vi "ReserveMemory.vi"(8 "error in (no error)":errorcluster, 10 "#DGs":i32=1, 11 "BME_DG_System in":refnum<class "BME_DG_System.lvclass">) -> (0 "error out":errorcluster, 3 "BME_DG_System out":refnum<class "BME_DG_System.lvclass">)   [LabVIEW 2009, in "BME_DG_System.lvclass"]
uses:
  BME_DG_System.lvclass
  BME_DG_System.lvclass/BME_DG_System.ctl
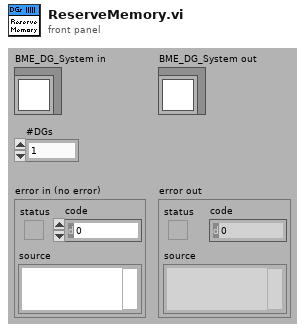
[diagram p1: front panel]
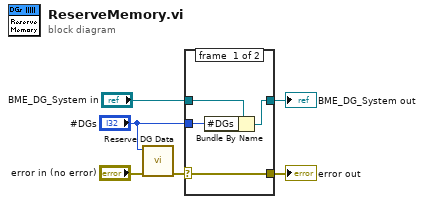
[diagram p0: block diagram]
diagram:
  n1 = call "Reserve DG Data.vi"("error in (no error)"="error in (no error)", "Number Of Delay Generators"="#DGs") -> ("error out"=w1:errorcluster)  [unwired: 9 in]
  n2 = case shown="No Error" w1 {
    selector: w1 -> [w9 w12]
    tunnel: [w9 w12] -> w6
    tunnel: [w8 w11] -> w4
    tunnel: "BME_DG_System in" -> [w10 w11]
    tunnel: "#DGs" -> [w7 _]
    frame #0 {
      n3 = Bundle By Name(cluster=w10, "#DGs"=w7) -> (w8:refnum<class "BME_DG_System.lvclass">)
    }
    frame #1 {
    }
  }
  "error out" <- w6
  "BME_DG_System out" <- w4
